vi "Activation Conditions.vi"(11 "App Data":T1={"Pump Station Controls"={"Lag Pump"=enum."OFF", "Lead Pump"=enum."OFF", "ALARM"=0.0, "LAG"=0.0, "LEAD"=0.0, "STOP"=0.0}, "Pump Indicators"={"Pump Water Level"=0.0, "ALARM"=FALSE, "LAG"=FALSE, "LEAD"=FALSE, "STOP"=FALSE, "PUMP 1 STATE"=FALSE, "PUMP 2 STATE"=FALSE}, "Alarm"=refnum, "Lag Start Time"=timestamp(0 s since 1904-01-01), "Lead Start Time"=timestamp(0 s since 1904-01-01), "Main Q"=refnum} {"Pump Indicators"."Pump Water Level" scale=0.0..4.0}) -> (3 "App Data 2":T1={"Pump Station Controls"={"Lag Pump"=enum."OFF", "Lead Pump"=enum."OFF", "ALARM"=0.0, "LAG"=0.0, "LEAD"=0.0, "STOP"=0.0}, "Pump Indicators"={"Pump Water Level"=0.0, "ALARM"=FALSE, "LAG"=FALSE, "LEAD"=FALSE, "STOP"=FALSE, "PUMP 1 STATE"=FALSE, "PUMP 2 STATE"=FALSE}, "Alarm"=refnum, "Lag Start Time"=timestamp(0 s since 1904-01-01), "Lead Start Time"=timestamp(0 s since 1904-01-01), "Main Q"=refnum} {"Pump Indicators"."Pump Water Level" scale=0.0..4.0})   [LabVIEW 2024]
uses:
  App Data.ctl
  Pump Controls.ctl
  Pump Switch.ctl
  Pump Indicators.ctl
  Q Info.ctl
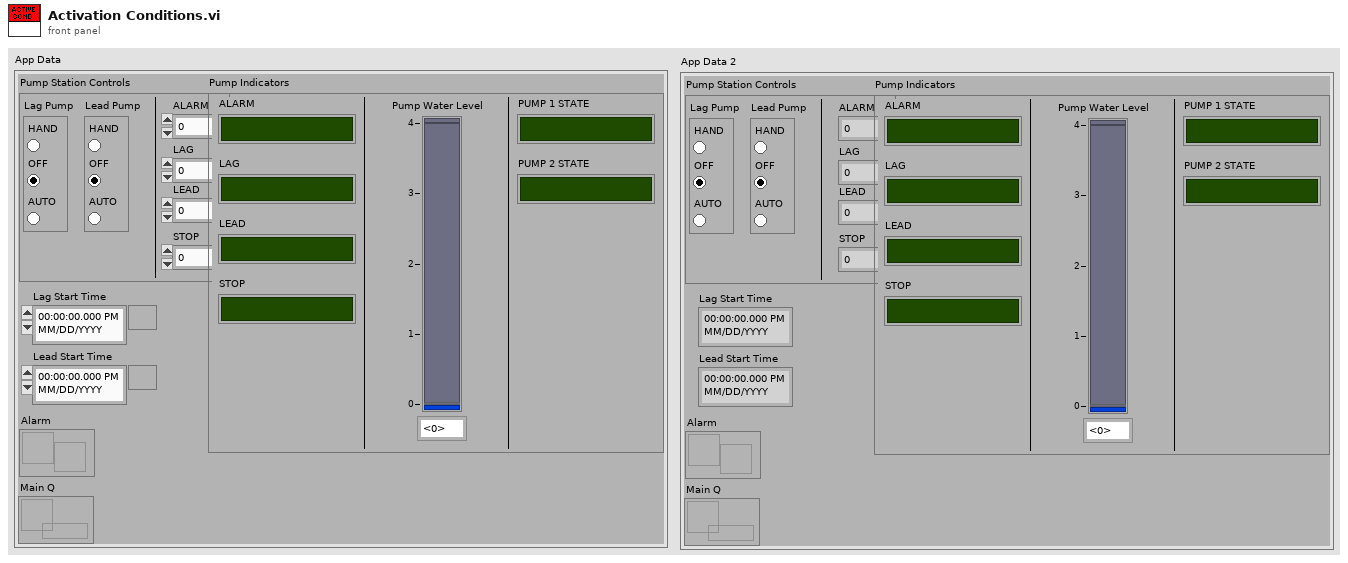
[diagram p1: front panel]
types:
  T1 = typedef "App Data.ctl" = cluster{"Pump Station Controls":T2, "Pump Indicators":T4, "Alarm":refnum<notifier>, "Lag Start Time":timestamp, "Lead Start Time":timestamp, "Main Q":refnum<queue>}
  T2 = typedef "Pump Controls.ctl" = cluster{"Lag Pump":T3, "Lead Pump":T3, "ALARM":dbl, "LAG":dbl, "LEAD":dbl, "STOP":dbl}
  T3 = typedef "Pump Switch.ctl" = enum32{"HAND", "OFF", "AUTO"}
  T4 = typedef "Pump Indicators.ctl" = cluster{"Pump Water Level":dbl, "ALARM":bool, "LAG":bool, "LEAD":bool, "STOP":bool, "PUMP 1 STATE":bool, "PUMP 2 STATE":bool}
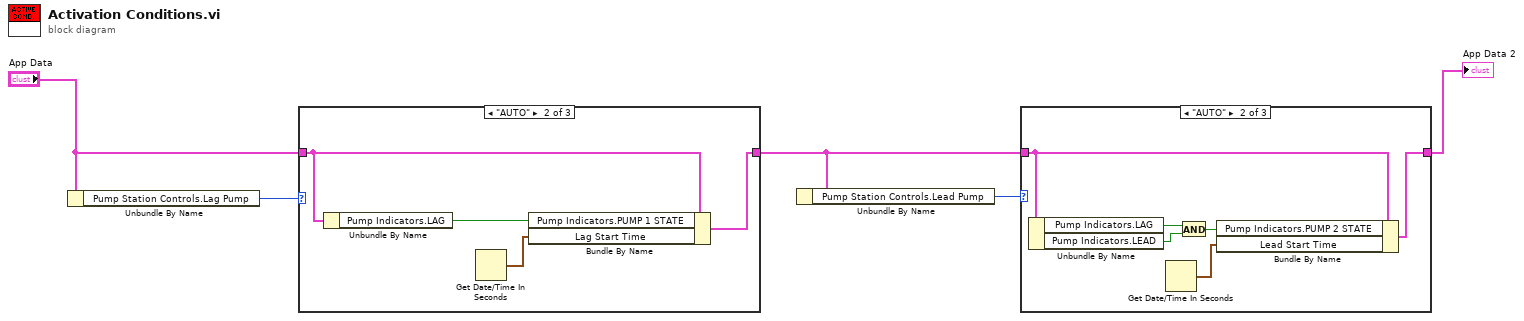
[diagram p0: block diagram]
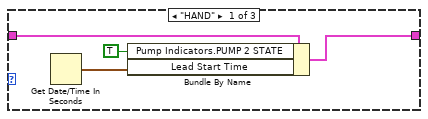
[diagram p2: hidden frame]
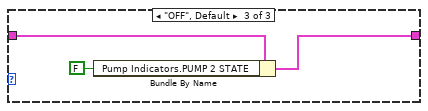
[diagram p3: hidden frame]
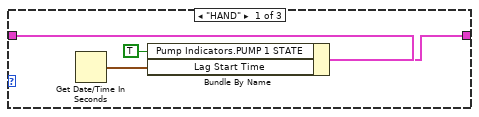
[diagram p4: hidden frame]
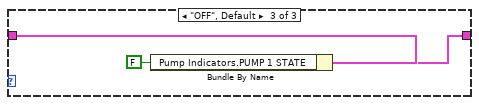
[diagram p5: hidden frame]
diagram:
  n1 = Unbundle By Name("App Data") -> ("Pump Station Controls.Lag Pump"=w2:T3)
  n2 = case shown="\"AUTO\"" w2 {
    tunnel: "App Data" -> [w9 w13 w16]
    tunnel: [w8 w12 w14] -> w4
    frame "HAND" {
      n3 = Get Date/Time In Seconds() -> (seconds since 1Jan1904=w6:timestamp)
      n4 = Bundle By Name(cluster=w9, "Pump Indicators.PUMP 1 STATE"=TRUE, "Lag Start Time"=w6) -> (w8:T1)
    }
    frame "AUTO" {
      n5 = Unbundle By Name(w13) -> ("Pump Indicators.LAG"=w11:bool)
      n6 = Get Date/Time In Seconds() -> (seconds since 1Jan1904=w10:timestamp)
      n7 = Bundle By Name(cluster=w13, "Pump Indicators.PUMP 1 STATE"=w11, "Lag Start Time"=w10) -> (w12:T1)
    }
    frame "OFF", Default {
      n8 = Bundle By Name(cluster=w16, "Pump Indicators.PUMP 1 STATE"=FALSE) -> (w14:T1)
    }
  }
  n9 = Unbundle By Name(w4) -> ("Pump Station Controls.Lead Pump"=w1:T3)
  n10 = case shown="\"AUTO\"" w1 {
    tunnel: w4 -> [w20 w24 w29]
    tunnel: [w19 w22 w27] -> w3
    frame "HAND" {
      n11 = Get Date/Time In Seconds() -> (seconds since 1Jan1904=w17:timestamp)
      n12 = Bundle By Name(cluster=w20, "Pump Indicators.PUMP 2 STATE"=TRUE, "Lead Start Time"=w17) -> (w19:T1)
    }
    frame "AUTO" {
      n13 = Unbundle By Name(w24) -> ("Pump Indicators.LAG"=w26:bool, "Pump Indicators.LEAD"=w25:bool)
      n14 = Get Date/Time In Seconds() -> (seconds since 1Jan1904=w21:timestamp)
      n15 = And(x=w26, y=w25) -> (x .and. y?=w23:bool)
      n16 = Bundle By Name(cluster=w24, "Pump Indicators.PUMP 2 STATE"=w23, "Lead Start Time"=w21) -> (w22:T1)
    }
    frame "OFF", Default {
      n17 = Bundle By Name(cluster=w29, "Pump Indicators.PUMP 2 STATE"=FALSE) -> (w27:T1)
    }
  }
  "App Data 2" <- w3
